vi "PSDATA_Variant To Bool.vi"(9 "error in":errorcluster, 10 "Value":variant) -> (1 "error out":errorcluster, 2 "Value":string, 4 "Bool":bool)   [LabVIEW 2016]
doc: "Developer：YDX"
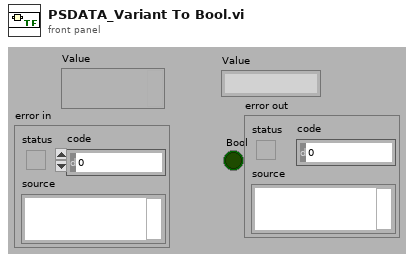
[diagram p1: front panel]
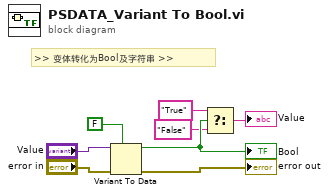
[diagram p0: block diagram]
diagram:
  # ">> 变体转化为Bool及字符串 >>"
  n1 = Variant To Data(error in="error in", type=FALSE ("Str"), Variant="Value") -> (data=w3:bool, error out=→"error out":errorcluster)
  "Bool" <- w3
  n2 = Select(t="True" ("y"), s=w3, f="False") -> (s? t:f=→"Value":string)
